vi "Read position.vi"(8 "error in (no error)":errorcluster, 11 "Shield in":refnum<class "Shield.lvclass">) -> (0 "error out":errorcluster, 2 "position":cluster{"x":dbl, "y":dbl}, 3 "Shield out":refnum<class "Shield.lvclass">)   [LabVIEW 2021]
uses:
  Shield.lvclass
  C:/Users/poche/Programs/LabVIEW/Snake Game/GameEl_class/GameEl.lvclass
  C:/Users/poche/Programs/LabVIEW/Snake Game/Shield/Shield.lvclass
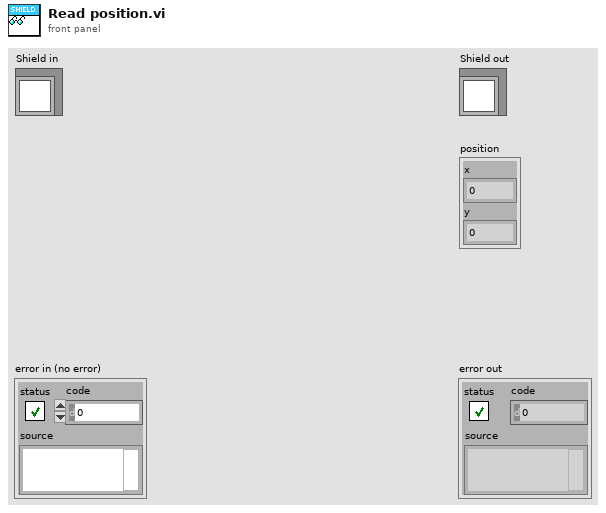
[diagram p1: front panel]
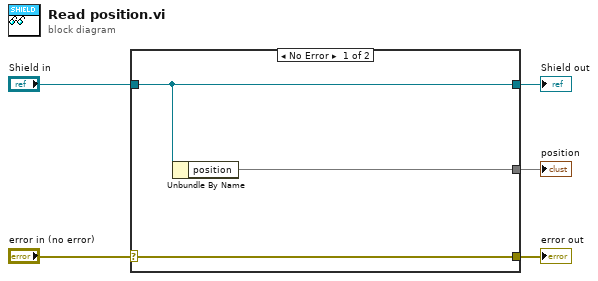
[diagram p0: block diagram]
diagram:
  n1 = case shown="No Error" "error in (no error)" {
    selector: "error in (no error)" -> [w8 w9]
    tunnel: [w8 w9] -> w4
    tunnel: [w7 w10] -> w2
    tunnel: "Shield in" -> [w7 w10]
    tunnel: [w6 _] -> w1
    frame No Error {
      n2 = Unbundle By Name(w7) -> ("position"=w6)
    }
    frame Error {
    }
  }
  "error out" <- w4
  "Shield out" <- w2
  "position" <- w1
